vi "GetState.vi"(11 "DriveBase in":refnum<class "DriveBase.lvclass">) -> (2 "State":T1, 3 "DriveBase out":refnum<class "DriveBase.lvclass">)   [LabVIEW 2016, in "DriveBase.lvclass"]
uses:
  DriveBase.lvclass
  DriveStates.ctl
  DriveBase.lvclass/DriveBase.ctl
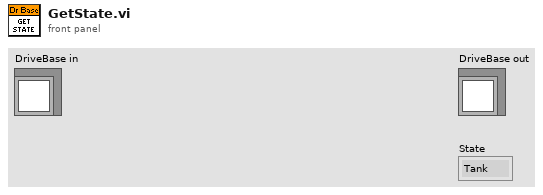
[diagram p1: front panel]
types:
  T1 = typedef "DriveBase.lvclass/DriveStates.ctl" = enum16{"Tank", "Arcade", "DriveStraight"}
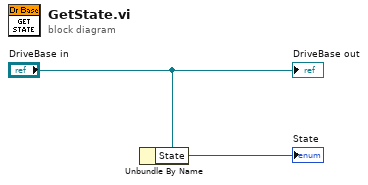
[diagram p0: block diagram]
diagram:
  n1 = Unbundle By Name("DriveBase in") -> ("State"=→"State":T1)
  "DriveBase out" <- "DriveBase in"
